vi "frontPanel.vi"(8 "error in (no error)":errorcluster, 10 "ScriptEvent":refnum<class "ScriptEvent.lvclass">, 11 "ActionPanel in":refnum<class "playFileAction.lvclass">) -> (0 "error out":errorcluster, 2 "ScriptEvent out":refnum<class "ScriptEvent.lvclass">, 3 "ActionPanel out":refnum<class "playFileAction.lvclass">)   [LabVIEW 2011, in "Views.lvlib" / "ScriptEditor.lvlib" / "playFileAction.lvclass"]
uses:
  playFileAction.lvclass
  Tools/Scripting/ScriptingEvent/ScriptEvent.lvclass
  playFileAction.lvclass/playFileAction.ctl
  Tools/Filing/FileSystem/FileSystem.lvclass
  ActionPanel.lvclass
panel:
  in  "Browse":bool
  in  "filePath":string
  out "Value":string caption="First Value"
  in  "Dt":dbl
  in  "Time":dbl
  out "Time Length":dbl
  out "ready?":bool
  out "editing":bool
  in  "close":bool
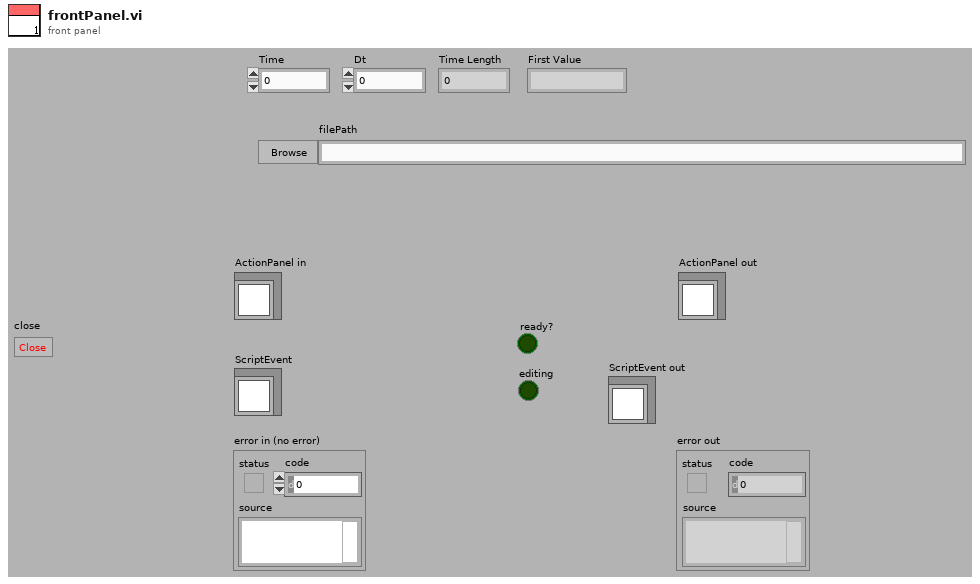
[diagram p1: front panel]
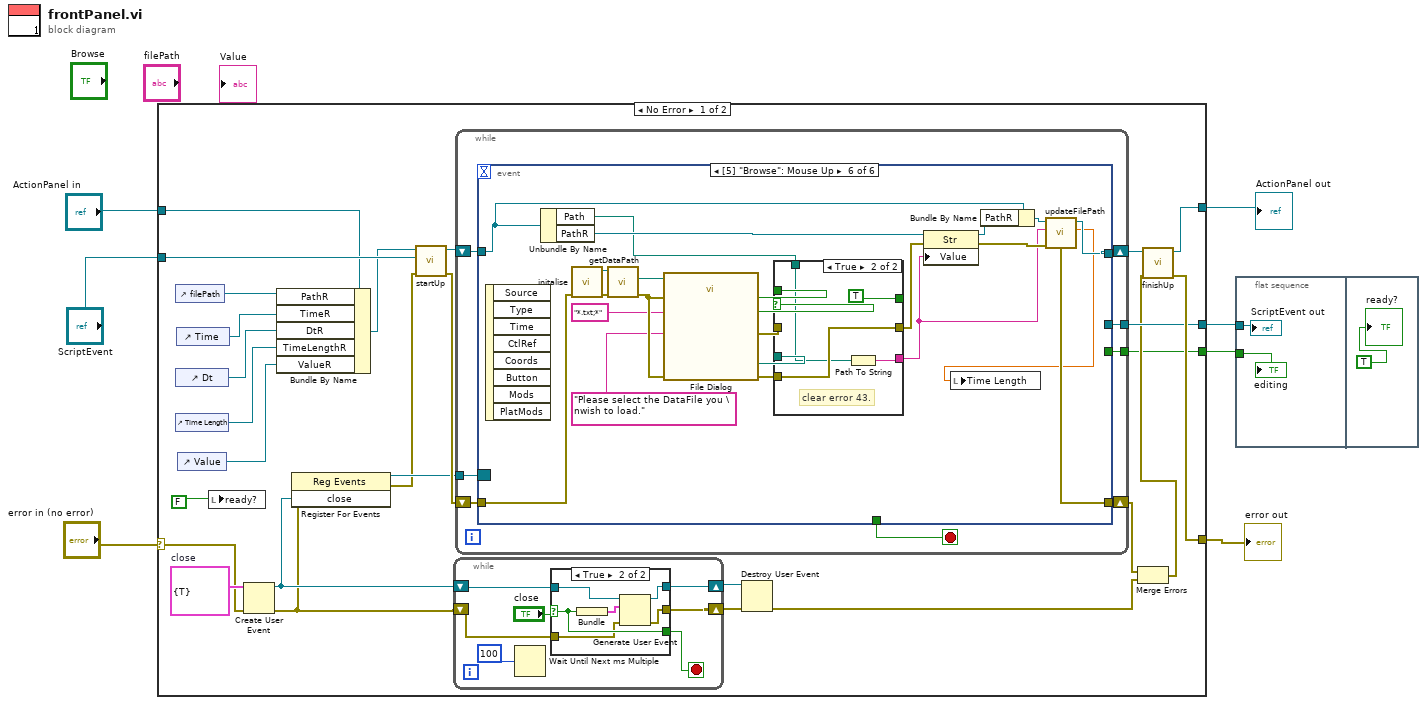
[diagram p0: block diagram]
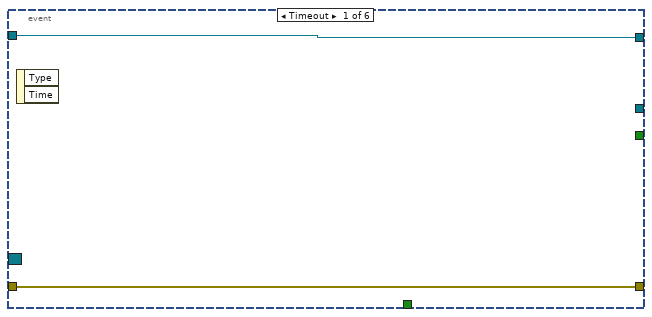
[diagram p3: hidden frame]
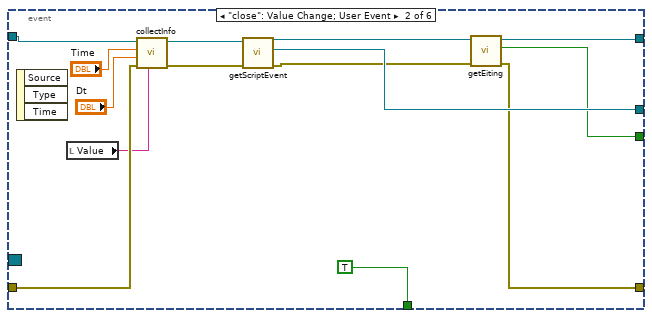
[diagram p4: hidden frame]
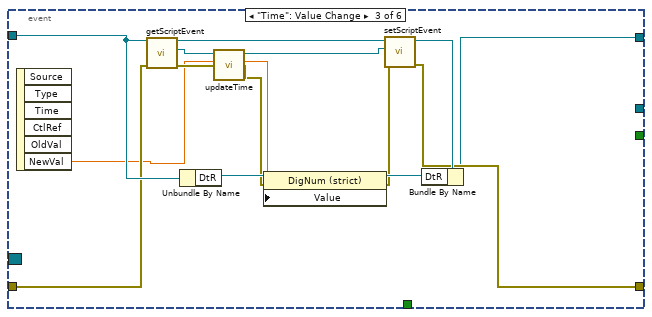
[diagram p5: hidden frame]
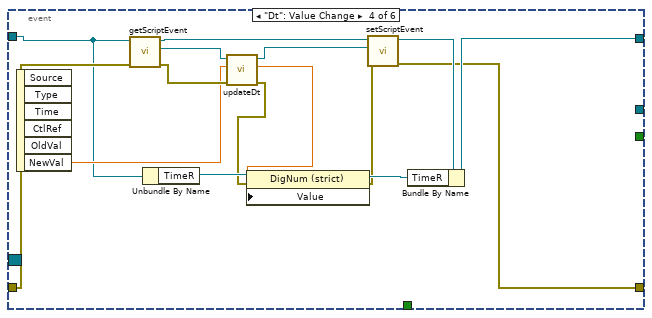
[diagram p6: hidden frame]
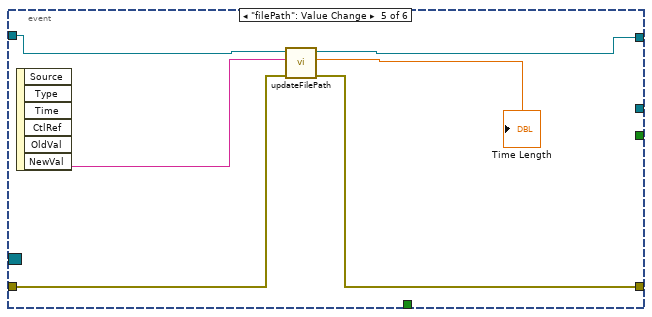
[diagram p7: hidden frame]
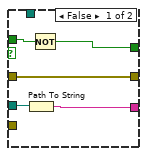
[diagram p8: hidden frame]
diagram:
  n1 = case shown="No Error" "error in (no error)" {
    selector: "error in (no error)" -> [w25 w142]
    tunnel: "ActionPanel in" -> [w14 w143]
    tunnel: [w29 w142] -> w4
    tunnel: [w30 w143] -> w5
    tunnel: "ScriptEvent" -> [w33 _]
    tunnel: [w27 _] -> w7
    tunnel: [w15 _] -> w6
    frame No Error {
      w26 = cluster{"close":bool} {"close"=TRUE}  # close
      n2 = control-ref of="filePath"() -> (w8:refnum<vi>)
      n3 = control-ref of="Dt"() -> (w11:refnum<vi>)
      n4 = control-ref of="Time Length"() -> (w10:refnum<vi>)
      n5 = control-ref of="Time"() -> (w12:refnum<vi>)
      n6 = control-ref of="Value"() -> (w9:refnum<vi>)
      n7 = local write "ready?"(FALSE) -> ()
      n8 = Create User Event(user event datatype=w26, error in=w25) -> (user event=w23:refnum<user-event>, error out=w20:errorcluster)
      n9 = Bundle By Name(cluster=w14, "PathR"=w8, "TimeR"=w12, "DtR"=w11, "TimeLengthR"=w10, "ValueR"=w9) -> (w13:refnum<class "playFileAction.lvclass">)
      n10 = register-events(error in=w20, w23) -> (reference out=w24:refnum<event-registration>, error out=w16:errorcluster)  [unwired: 1 in]
      n11 = call-dynamic "startUp.vi"("error in (no error)"=w16, "ScriptEvent"=w33, "playFileAction in"=w13) -> ("error out"=w32:errorcluster, "playFileAction out"=w34:refnum<class "playFileAction.lvclass">)  [unwired: 7 in]
      n12 = while {
        shift-right: [w37] -> w21
        shift-left: w20 -> [w36]
        shift-right: [w38] -> w22
        shift-left: w23 -> [w41]
        stop <- w39 stop-if-true
        n13 = Wait Until Next ms Multiple(millisecond multiple=100) -> ()  [unwired: 1 out]
        n14 = case shown="True" "close" {
          selector: "close" -> [w44 w48]
          tunnel: w41 -> [w43 w50]
          tunnel: [w44 w48] -> w39
          tunnel: [w43 w47] -> w38
          tunnel: [w42 w46] -> w37
          tunnel: w36 -> [w42 w45]
          frame False {
          }
          frame True {
            n15 = Bundle(w48) -> (w49:cluster{bool})  [unwired: 1 in]
            n16 = Generate User Event(user event=w50, event data cluster=w49, error in=w45) -> (user event out=w47:refnum<user-event>, error out=w46:errorcluster)
          }
        }
      }
      n17 = while {
        shift-right: [w58] -> w31
        shift-left: w34 -> [w57]
        shift-right: [w55] -> w19
        shift-left: w32 -> [w56]
        tunnel: [w53] -> w27
        tunnel: w24 -> [w52]
        tunnel: [w51] -> w15
        stop <- w54 stop-if-true
        n18 = event shown="[5] \"Browse\": Mouse Up" {
          selector: w52 -> [_ _ _ _ _ _]
          dyn-events: _ -> [_ _ _ _ _ _]
          timeout: _ -> [_ _ _ _ _ _]
          tunnel: [w60 w71 w75 w91 w109 w115] -> w58
          tunnel: w57 -> [w60 w66 w79 w94 w110 w117]
          tunnel: [w59 w69 w76 w90 w106 w112] -> w55
          tunnel: w56 -> [w59 w65 w78 w96 w107 w123]
          tunnel: [_ TRUE _ _ _ _] -> w54
          tunnel: [_ w74 _ _ _ _] -> w53
          tunnel: [_ w68 _ _ _ _] -> w51
          event Timeout {
            n19 = event-data() -> ()  [unwired: 1 in, 2 out]
          }
          event "close": Value Change; User Event {
            n20 = event-data() -> ()  [unwired: 1 in, 3 out]
            n21 = local read "Value"() -> (w61:string)
            n22 = call "collectInfo.vi"("Value"=w61, "error in (no error)"=w65, "Dt"="Dt", "Time"="Time", "playFileAction in"=w66) -> ("error out"=w64:errorcluster, "playFileAction out"=w67:refnum<class "playFileAction.lvclass">)  [unwired: 5 in]
            n23 = call "getScriptEvent.vi"("error in (no error)"=w64, "ActionPanel.lvclass in"=w67) -> ("error out"=w70:errorcluster, "ScriptEvent.lvclass"=w74:refnum<class "ScriptEvent.lvclass">, "ActionPanel.lvclass out"=w72:refnum<class "playFileAction.lvclass">)  [unwired: 7 in]
            n24 = call "getEiting.vi"("error in (no error)"=w70, "ActionPanel.lvclass in"=w72) -> ("error out"=w69:errorcluster, "editing?"=w68:bool, "ActionPanel.lvclass out"=w71:refnum<class "playFileAction.lvclass">)  [unwired: 7 in]
          }
          event "Time": Value Change {
            n25 = event-data() -> ("NewVal"=w77:dbl)  [unwired: 1 in, 5 out]
            n26 = call "getScriptEvent.vi"("error in (no error)"=w78, "ActionPanel.lvclass in"=w79) -> ("error out"=w87:errorcluster, "ScriptEvent.lvclass"=w88:refnum<class "ScriptEvent.lvclass">, "ActionPanel.lvclass out"=w89:refnum<class "playFileAction.lvclass">)  [unwired: 7 in]
            n27 = Unbundle By Name(w79) -> ("DtR"=w86:refnum<vi>)
            n28 = call "updateTime.vi"("error in (no error)"=w87, "time"=w77, "ScriptEvent in"=w88) -> ("error out"=w85:errorcluster, "dt"=w84:dbl, "ScriptEvent out"=w80:refnum<class "ScriptEvent.lvclass">)  [unwired: 6 in]
            n29 = property class="DigNum (strict)"(reference=w86, error in=w85, "Value"=w84) -> (reference out=w83:refnum<vi>, error out=w81:errorcluster)
            n30 = call "setScriptEvent.vi"("error in (no error)"=w81, "ScriptEvent.lvclass"=w80, "ActionPanel.lvclass in"=w89) -> ("error out"=w76:errorcluster, "ActionPanel.lvclass out"=w82:refnum<class "playFileAction.lvclass">)  [unwired: 7 in]
            n31 = Bundle By Name(cluster=w82, "DtR"=w83) -> (w75:refnum<class "playFileAction.lvclass">)
          }
          event "Dt": Value Change {
            n32 = event-data() -> ("NewVal"=w95:dbl)  [unwired: 1 in, 5 out]
            n33 = call "getScriptEvent.vi"("error in (no error)"=w96, "ActionPanel.lvclass in"=w94) -> ("error out"=w100:errorcluster, "ScriptEvent.lvclass"=w101:refnum<class "ScriptEvent.lvclass">, "ActionPanel.lvclass out"=w93:refnum<class "playFileAction.lvclass">)  [unwired: 7 in]
            n34 = Unbundle By Name(w94) -> ("TimeR"=w104:refnum<vi>)
            n35 = call "updateDt.vi"("error in (no error)"=w100, "dt"=w95, "ScriptEvent in"=w101) -> ("error out"=w98:errorcluster, "time"=w99:dbl, "ScriptEvent out"=w97:refnum<class "ScriptEvent.lvclass">)  [unwired: 6 in]
            n36 = property class="DigNum (strict)"(reference=w104, error in=w98, "Value"=w99) -> (reference out=w103:refnum<vi>, error out=w102:errorcluster)
            n37 = call "setScriptEvent.vi"("error in (no error)"=w102, "ScriptEvent.lvclass"=w97, "ActionPanel.lvclass in"=w93) -> ("error out"=w90:errorcluster, "ActionPanel.lvclass out"=w92:refnum<class "playFileAction.lvclass">)  [unwired: 7 in]
            n38 = Bundle By Name(cluster=w92, "TimeR"=w103) -> (w91:refnum<class "playFileAction.lvclass">)
          }
          event "filePath": Value Change {
            n39 = event-data() -> ("NewVal"=w108:string)  [unwired: 1 in, 5 out]
            n40 = call "updateFilePath.vi"("error in (no error)"=w107, "path"=w108, "playFileAction in"=w110) -> ("error out"=w106:errorcluster, "timeLength"=→"Time Length":dbl, "playFileAction out"=w109:refnum<class "playFileAction.lvclass">)  [unwired: 6 in]
          }
          event "Browse": Mouse Up {
            n41 = event-data() -> ()  [unwired: 1 in, 8 out]
            n42 = Unbundle By Name(w117) -> ("Path"=w120:path, "PathR"=w121:refnum<vi>)
            n43 = call "initalise.vi"("error in (no error)"=w123) -> ("error out"=w126:errorcluster, "FileSystem out"=w125:refnum<class "FileSystem.lvclass">)  [unwired: 9 in]
            n44 = call-dynamic "getDataPath.vi"("error in (no error)"=w126, "FileSystem.lvclass in"=w125) -> ("error out"=w132:errorcluster, "DataPath"=w124:path)  [unwired: 7 in, 1 out]
            n45 = call "File Dialog"("start path"=w124, "prompt"="Please select the DataFile you \nwish to load.", "error in"=w132, "pattern (all files)"="*.txt;*") -> ("selected path"=w122:path, "exists"=w130:bool, "cancelled"=w129:bool, "error out"=w131:errorcluster)  [unwired: 8 in]
            n46 = case shown="True" w129 {
              tunnel: [w136 TRUE] -> _
              tunnel: w130 -> [w137 _]
              tunnel: w131 -> [w135 _]
              tunnel: [w135 w140] -> w119
              tunnel: w132 -> [_ w140]
              tunnel: w122 -> [w134 _]
              tunnel: [w133 w139] -> w113
              tunnel: w120 -> [_ w138]
              frame False {
                n47 = Path To String(path=w134) -> (string=w133:string)
                n48 = Not(x=w137) -> (.not. x?=w136:bool)
              }
              frame True {
                # "clear error 43."
                n49 = Path To String(path=w138) -> (string=w139:string)
              }
            }
            n50 = property class="Str"(reference=w121, error in=w119, "Value"=w113) -> (reference out=w118:refnum<vi>, error out=w114:errorcluster)
            n51 = Bundle By Name(cluster=w117, "PathR"=w118) -> (w116:refnum<class "playFileAction.lvclass">)
            n52 = call "updateFilePath.vi"("error in (no error)"=w114, "path"=w113, "playFileAction in"=w116) -> ("error out"=w112:errorcluster, "timeLength"=w111:dbl, "playFileAction out"=w115:refnum<class "playFileAction.lvclass">)  [unwired: 6 in]
            n53 = local write "Time Length"(w111) -> ()
          }
        }
      }
      n54 = Destroy User Event(user event=w22, error in=w21) -> (error out=w17:errorcluster)
      n55 = Merge Errors(w19, w17) -> (w18:errorcluster)
      n56 = call-dynamic "finishUp.vi"("error in (no error)"=w18, "ActionPanel in"=w31) -> ("error out"=w29:errorcluster, "ActionPanel out"=w30:refnum<class "playFileAction.lvclass">)  [unwired: 8 in]
    }
    frame Error {
    }
  }
  "error out" <- w4
  "ActionPanel out" <- w5
  n57 = flat-sequence {
    tunnel: w7 -> [w145]
    tunnel: w6 -> [w144]
    frame #0 {
      "ScriptEvent out" <- w145
      "editing" <- w144
    }
    frame #1 {
      "ready?" <- TRUE
    }
  }
